vi "Release.vi"(8 "error in (no error)":errorcluster, 11 "CLILogger in":refnum<class "CLILogger.lvclass">) -> (0 "error out":errorcluster)   [LabVIEW 2020, in "GPackTools.lvlib" / "CLILogger.lvclass"]
uses:
  CLILogger.lvclass
  CLILogger.lvclass/CLILogger.ctl
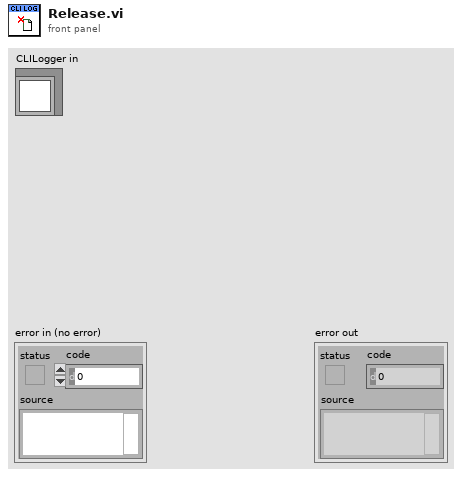
[diagram p1: front panel]
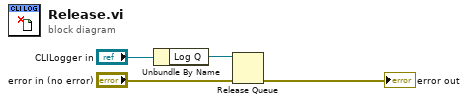
[diagram p0: block diagram]
diagram:
  n1 = Unbundle By Name("CLILogger in") -> ("Log Q"=w2:refnum<queue>)
  n2 = Release Queue(queue=w2, error in (no error)="error in (no error)") -> (error out=→"error out":errorcluster)  [unwired: 1 in, 2 out]
